vi "Install.vi"   [LabVIEW 2013]
uses:
  ClassMethodsInheritance/ClassMethodsInheritance.lvclass
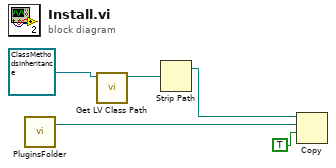
[diagram p0: block diagram]
diagram:
  n1 = call <resource>:"PluginsFolder.vi"() -> ("PluginsFolderPath"=w5:path)  [unwired: 3 in]
  n2 = call <vilib>:"Get LV Class Path.vi"("object"=refnum<class "ClassMethodsInheritance.lvclass"> refnum ("ClassMethodsInheritance")) -> ("class path"=w3:path)  [unwired: 9 in, 1 out]
  n3 = Strip Path(path=w3) -> (stripped path=w2:path)  [unwired: 1 out]
  n4 = Copy(9:TRUE ("overwrite (F)"), 10:w5, 11:w2) -> ()  [unwired: 2 in, 3 out]
